vi "In-Context Exit Set Actions-Rev5.vi"(0 "Acquisition Parameters In":T5={"Magnet Angle [deg]"=0.0, "Magnet Angles [deg]"=[], "DeltaVpp [v]"=0.0, "SEM [v]"=0.0, "DeltaVpp Thresh [v]"=0.0, "SEM Thresh [v]"=0.0, "Adaptive Processing"=FALSE, "Acquire Q"=FALSE, "Acquire Photos"=FALSE, "Adaptive Tuning"=FALSE, "Automated Matching"=FALSE, "X-Gradient [G/mm]"=0.0, "Y-Gradient [G/mm]"=0.0, "Z-Gradient [G/mm]"=0.0, "Central Field [G]"=0.0, "Scan Width [G]"=0.0, "Mod. Amp. [G]"=0.0, "Scan Time [s]"=0.0, "Pre-Scan Delay [ms]"=0, "Measurement Timeout [s]"=0.0, "Electromagnet Main Field [G]"=0.0, "Locked Central Field [G]"=0.0, "Scans Excluded"=0, "Scans Completed"=0, "No. Scans/Set"=0, "No. Scans for SNR"=0, "Field Locked Frequency [GHz]"=0.0, "Auto Set-based Field Center"=FALSE, "Prompt for oxy acquisition updates"=FALSE, "Oxy QA Scan?"=FALSE, "Exclude Bad Data"=FALSE, "Optimizing RF Power"=FALSE, "Gradients on/off"=TRUE, "Running Script"=FALSE, "Opto-Coupler Current [A]"=0.0, "Continuous Sweeping"=FALSE, "Sweep Rise Time [sec]"=0, "Reverse Sweep Central Field [G]"=0.0, "Forward Sweep Central Field [G]"=0.0, "Sweep Calibrated"=FALSE, "Modulation Calibrated"=FALSE, "First CheckCal Scan?"=FALSE, "AFC Field Correction"=FALSE, "OxyQAInit Scan Width [G]"=0.0, "OxyQAInit Mod. Amp. [G]"=0.0, "Scans Completed/Session"=0, "Acquire SpO2"=FALSE, "Acquire Temperature"=FALSE, "Over Mod"=FALSE} {"OxyQAInit Mod. Amp. [G]" min=0.0; "OxyQAInit Scan Width [G]" min=0.0; "Mod. Amp. [G]" min=0.0; "Scan Width [G]" min=0.0; "Measurement Timeout [s]" min=0.0; "Scan Time [s]" min=0.0; "Z-Gradient [G/mm]" min=0.0; "Y-Gradient [G/mm]" min=0.0; "X-Gradient [G/mm]" min=0.0; "SEM Thresh [v]" min=0.0; "DeltaVpp Thresh [v]" min=0.0; "SEM [v]" min=0.0}, 5 "Hardware Parameters In":T8={"Scan Calibration [G/V]"=0.0, "Modulation Calibration [G/V]"=0.0, "Modulation Phase [deg]"=0.0, "Modulation Frequency [Hz]"=0.0, "Attenuation [dB]"=0, "Input Channel Count"=0, "Time constant"=7, "Sensitivity"=17, "Frequency Output Voltage [V]"=0.0, "Phase Output Voltage [V]"=0.0, "Lock-in Offset Compensation"=FALSE, "RF [GHz]"=0.0, "Q Start"=0.0, "Q End"=0.0, "Balance"=0.0, "Phase Error"=0.0, "AFC Error"=0.0, "AFC"=FALSE, "Magnet Rotation"=FALSE, "Balance Scaling Factor"=1.0, "Phase Error Scaling Factor"=1.0, "AFC Error Scaling Factor"=1.0, "Frequency Counter ID"="", "Sweep Waveform"=enum."Sawtooth", "Q-Factor Scale"=0.0, " Q-Data Scale"=0.0, " Q-Data Offset"=0.0, "Magnet Rotation Slope"=0.0, "Magnet Rotation Offset"=0.0, "Phase Sweep Resolution"=0.0, "Hardware Version Number"="", "Spectrometer ID Number"=0, "Spectrometer Name"="", "Lock in Saturation"=0.0, "Balance Threshold"=0.0, "Phase Error Threshold"=0.0, "AFC Error Threshold"=0.0, "Linear Actuator Length"=0.0, "Lock-in OK?"=FALSE, "Ignore Lock-in Comm. Failure"=FALSE, "Gradient Addresses"=[], "Gradient Calibrations [G/A*mm]"=[], "Gradient Power Supplies"=[], "Lock-in Address"="", "Magnet Type"=enum."RRI", "Camera Names"=[], "Sweep Limit [Gauss]"=0.0, "Modulation Limit [Gauss]"=0.0, "Balance Threshold Exceeded?"=FALSE, "Phase Threshold Exceeded?"=FALSE, "AFC Threshold Exceeded?"=FALSE, "Consecutive Re-tune attempts"=0, "Reverse Sweep Slope [sec]"=0.0, "Reverse Sweep Offset [G]"=0.0, "AFC Field Correction [V/MHz]"=0.0, "Active Gradients (X Y Z)"=[], "SpO2 Calibration [SpO2/V]"=1.0, "Heart Rate Calibration [BPM/V]"=1.0, "Thermocouple Channel"=""} {"Sensitivity" items=["", "2 nV", "5 nV", "10 nV", "20 nV", "50 nV", "100 nV", "200 nV", "500 nV", "1 uV", "2 uV", "5 uV", "10 uV", "20 uV", "50 uV", "100 uV", "200 uV", "500 uV", "1 mV", "2 mV", "5 mV", "10 mV", "20 mV", "50 mV", "100 mV", "200 mV", "500 mV", "1 V"]; "Time constant" items=["10 us", "20 us", "40 us", "80 us", "160 us", "320 us", "640 us", "5 ms", "10 ms", "20 ms", "50 ms", "100 ms", "200 ms", "500 ms", "1 s", "2 s", "5 s", "10 s", "20 s", "50 s", "100 s", "200 s", "500 s", "1 ks", "2 ks", "5 ks", "10 ks", "20 ks", "50 ks", "100 ks"]}, 9 "Measurement Information In":T1={"Comments"="", "Directory Input"="", "Data file path"=path "C:/Data/EPR Data", "Scripting File"=path "C:/Data/Configuration Script.csv", "Save Data"=FALSE, "Tooth size (d11) [mm]"=0.0, "Tooth size (d12) [mm]"=0.0, "Tooth size (d21) [mm]"=0.0, "Tooth size (d22) [mm]"=0.0, "Dose of Tooth [Gy]"=0.0, "Safe Shutdown?"=FALSE, "Gases Available"=[], "Database Username"="", "Database Password"="", "Database Login URL"="", "Database Upload URL"="", "Database Success URL"="", "Database XML URL"="", "Database Resonator URL"="", "Session Number"=0, "Set #"=0, "Resonator Operator"="", "Session Type"="", "Tooth/Sample ID"="", "Volunteer ID"="", "Computer Operator"="", "Volunteer Type"="", "Site/Tooth Selection (T8,T9)"="", "Resonator"="", "Measurement Site"="", "Non-standard session?"=FALSE, "EPR DAQ Version"="", "Session Path"=path "C:/Data/EPR Data", "Chosen Applied State"="", "Chosen Initial State"="", "Time of Transition"="", "DAQ Mode"=enum."Engineering", "pO2/Scan [mmHg]"=[], "pO2/Set [mmHg]"=[], "Linewidth (HWHM)/Scan [Gauss]"=[], "Linewidth (HWHM)/Set [Gauss]"=[], "pO2 Conversion"="", "Dose Calibration Cluster"={"Dose Response"={"grand_mean"=0.0292016, "slope"=0.0188720543}, "Dose Correction"={"Sex"=1, "a0"=7.719669421, "a1"=-2.746550736, "a2"=-0.186490355, "a3"=0.041922063, "a4"=-0.849147359, "a5"=0.14330063, "a6"=0.019930219, "A_n"=40.0, "H_n"=10.12, "Dose Correction"=FALSE}, "Dose Reporting"={"Reporting is"=TRUE, "sd_threshold [AU]"=0.06, "sd_model [Gy]"=0.66, "dosimetric_threshold [Gy]"=2.0, "Add intrasession errors is"=FALSE, "Prior Radiation?"=FALSE}}, "OxyChip Slope"=0.0, "OxyChip Intercept"=0.0, "QA Mode"=enum."Select QA Mode", "QA Session?"=FALSE, "Sample Type"=enum."Empty Resonator", "Report pO2/Scan"=FALSE, "Skip End Session Save"=FALSE, "Number of sites"=enum."# Probes", "Recipient Name"="", "Sender Name"="", "Recipient Email"="", "Transition State History"=[], "pO2 Report Times"=[], "Temperature [C]"=0.0, "+Error pO2/Scan [mmHg]"=[], "-Error pO2/Scan [mmHg]"=[], "+Error pO2/Set [mmHg]"=[], "-Error pO2/Set [mmHg]"=[], "Oxy Phase Exclusion Tolerance [rad]"=0.0, "Oxy Center Exclusion Tolerance [%]"=0.0, "Oxy Exclude Unacceptable"=FALSE, "Oxy Unacceptable Estimate Flags"=[], "Save Session PPT"=FALSE, "Flagged Bad Sets"=[]} {"Oxy Center Exclusion Tolerance [%]" format="%#_9g"; "Oxy Phase Exclusion Tolerance [rad]" format="%#_9g"; "Temperature [C]" format="%#_9g"; "OxyChip Intercept" format="%#_9g"; "OxyChip Slope" format="%#_9g"; "Dose Calibration Cluster"."Dose Reporting"."dosimetric_threshold [Gy]" format="%#_9g"; "Dose Calibration Cluster"."Dose Reporting"."sd_model [Gy]" format="%#_9g"; "Dose Calibration Cluster"."Dose Reporting"."sd_threshold [AU]" format="%#_9g"; "Dose Calibration Cluster"."Dose Correction"."H_n" format="%#_9g"; "Dose Calibration Cluster"."Dose Correction"."A_n" format="%#_9g"; "Dose Calibration Cluster"."Dose Correction"."a6" format="%#.9g"; "Dose Calibration Cluster"."Dose Correction"."a5" format="%#.9g"; "Dose Calibration Cluster"."Dose Correction"."a4" format="%#.9g"; "Dose Calibration Cluster"."Dose Correction"."a3" format="%#.9g"; "Dose Calibration Cluster"."Dose Correction"."a2" format="%#.9g"; "Dose Calibration Cluster"."Dose Correction"."a1" format="%#.9g"; "Dose Calibration Cluster"."Dose Correction"."a0" format="%#.9g"; "Dose Calibration Cluster"."Dose Correction"."Sex" items=["Male"=1, "Female"=0]; "Dose Calibration Cluster"."Dose Response"."slope" format="%#_9g"; "Dose Calibration Cluster"."Dose Response"."grand_mean" format="%#_9g"}, 11 "Spectral Data In":T6={"PDT Amp [v]"=0.0, "RIS Amp [v]"=0.0, "B-Field"=[], "All In-Phase Scan Spectra"=[], "Model Select"=enum."OneCompRISTwoPDT", "Fit Each Scan"=FALSE, "PDT Center [g]"=0.0, "In-Phase Average Spectra"=[], "In-Phase Median Spectra"=[], "Out-Phase Median Spectra"=[], "Out-Phase Average Spectra"=[], "Fit Spectra"=[], "Fit No-Baseline Spectra"=[], "All Out-Phase Scan Spectra"=[], "Baseline Offset Correction"=FALSE, "In-Phase Offset [v]"=0.0, "Out-Phase Offset [v]"=0.0, "Ch2 Input\n(Balance)"=[], "Ch3 Input\n(Phase)"=[], "Ch4 Input\n(AFC)"=[], "Fit Pars"=[], "Fit Pars Errors"=[], "Fit Pars Labels"=[], "Raw Scan DAQ Data"=[], "Bad Scans Indicies"=[], "Good In-Phase Scan Spectra"=[], "Good Out-Phase Scan Spectra"=[], "Bad In-Phase Scan Spectra"=[], "Bad Out-Phase Scan Spectra"=[], "Number of bad scans"=0, "Fit History"=[], "PDT Amp. History/Set [v]"=[], "RIS Amp. History/Set [v]"=[], "RIS Amp. History/Scan [v]"=[], "All Shifted B-Fields"=[], "Good Shifted B-Fields"=[], "Ch5 Input\n(SpO2)"=[], "Ch6 Input\n(BPM)"=[], "Global SNR"=0.0, "Fit Error History"=[], "SNR History"=[]} {"Global SNR" min=0.0; "PDT Center [g]" min=0.0; "RIS Amp [v]" min=0.0; "PDT Amp [v]" min=0.0}) -> (1 "Exclude pO2 Estimate":bool, 2 "Scan Width [G]":dbl, 3 "Mod. Amp. [G]":dbl, 4 "Acquisition Parameters Out":T5={"Magnet Angle [deg]"=0.0, "Magnet Angles [deg]"=[], "DeltaVpp [v]"=0.0, "SEM [v]"=0.0, "DeltaVpp Thresh [v]"=0.0, "SEM Thresh [v]"=0.0, "Adaptive Processing"=FALSE, "Acquire Q"=FALSE, "Acquire Photos"=FALSE, "Adaptive Tuning"=FALSE, "Automated Matching"=FALSE, "X-Gradient [G/mm]"=0.0, "Y-Gradient [G/mm]"=0.0, "Z-Gradient [G/mm]"=0.0, "Central Field [G]"=0.0, "Scan Width [G]"=0.0, "Mod. Amp. [G]"=0.0, "Scan Time [s]"=0.0, "Pre-Scan Delay [ms]"=0, "Measurement Timeout [s]"=0.0, "Electromagnet Main Field [G]"=0.0, "Locked Central Field [G]"=0.0, "Scans Excluded"=0, "Scans Completed"=0, "No. Scans/Set"=0, "No. Scans for SNR"=0, "Field Locked Frequency [GHz]"=0.0, "Auto Set-based Field Center"=FALSE, "Prompt for oxy acquisition updates"=FALSE, "Oxy QA Scan?"=FALSE, "Exclude Bad Data"=FALSE, "Optimizing RF Power"=FALSE, "Gradients on/off"=TRUE, "Running Script"=FALSE, "Opto-Coupler Current [A]"=0.0, "Continuous Sweeping"=FALSE, "Sweep Rise Time [sec]"=0, "Reverse Sweep Central Field [G]"=0.0, "Forward Sweep Central Field [G]"=0.0, "Sweep Calibrated"=FALSE, "Modulation Calibrated"=FALSE, "First CheckCal Scan?"=FALSE, "AFC Field Correction"=FALSE, "OxyQAInit Scan Width [G]"=0.0, "OxyQAInit Mod. Amp. [G]"=0.0, "Scans Completed/Session"=0, "Acquire SpO2"=FALSE, "Acquire Temperature"=FALSE, "Over Mod"=FALSE} {"OxyQAInit Mod. Amp. [G]" min=0.0; "OxyQAInit Scan Width [G]" min=0.0; "Mod. Amp. [G]" min=0.0; "Scan Width [G]" min=0.0; "Measurement Timeout [s]" min=0.0; "Scan Time [s]" min=0.0; "Z-Gradient [G/mm]" min=0.0; "Y-Gradient [G/mm]" min=0.0; "X-Gradient [G/mm]" min=0.0; "SEM Thresh [v]" min=0.0; "DeltaVpp Thresh [v]" min=0.0; "SEM [v]" min=0.0}, 6 "Measurement Information Out":T1={"Comments"="", "Directory Input"="", "Data file path"=path "C:/Data/EPR Data", "Scripting File"=path "C:/Data/Configuration Script.csv", "Save Data"=FALSE, "Tooth size (d11) [mm]"=0.0, "Tooth size (d12) [mm]"=0.0, "Tooth size (d21) [mm]"=0.0, "Tooth size (d22) [mm]"=0.0, "Dose of Tooth [Gy]"=0.0, "Safe Shutdown?"=FALSE, "Gases Available"=[], "Database Username"="", "Database Password"="", "Database Login URL"="", "Database Upload URL"="", "Database Success URL"="", "Database XML URL"="", "Database Resonator URL"="", "Session Number"=0, "Set #"=0, "Resonator Operator"="", "Session Type"="", "Tooth/Sample ID"="", "Volunteer ID"="", "Computer Operator"="", "Volunteer Type"="", "Site/Tooth Selection (T8,T9)"="", "Resonator"="", "Measurement Site"="", "Non-standard session?"=FALSE, "EPR DAQ Version"="", "Session Path"=path "C:/Data/EPR Data", "Chosen Applied State"="", "Chosen Initial State"="", "Time of Transition"="", "DAQ Mode"=enum."Engineering", "pO2/Scan [mmHg]"=[], "pO2/Set [mmHg]"=[], "Linewidth (HWHM)/Scan [Gauss]"=[], "Linewidth (HWHM)/Set [Gauss]"=[], "pO2 Conversion"="", "Dose Calibration Cluster"={"Dose Response"={"grand_mean"=0.0292016, "slope"=0.0188720543}, "Dose Correction"={"Sex"=1, "a0"=7.719669421, "a1"=-2.746550736, "a2"=-0.186490355, "a3"=0.041922063, "a4"=-0.849147359, "a5"=0.14330063, "a6"=0.019930219, "A_n"=40.0, "H_n"=10.12, "Dose Correction"=FALSE}, "Dose Reporting"={"Reporting is"=TRUE, "sd_threshold [AU]"=0.06, "sd_model [Gy]"=0.66, "dosimetric_threshold [Gy]"=2.0, "Add intrasession errors is"=FALSE, "Prior Radiation?"=FALSE}}, "OxyChip Slope"=0.0, "OxyChip Intercept"=0.0, "QA Mode"=enum."Select QA Mode", "QA Session?"=FALSE, "Sample Type"=enum."Empty Resonator", "Report pO2/Scan"=FALSE, "Skip End Session Save"=FALSE, "Number of sites"=enum."# Probes", "Recipient Name"="", "Sender Name"="", "Recipient Email"="", "Transition State History"=[], "pO2 Report Times"=[], "Temperature [C]"=0.0, "+Error pO2/Scan [mmHg]"=[], "-Error pO2/Scan [mmHg]"=[], "+Error pO2/Set [mmHg]"=[], "-Error pO2/Set [mmHg]"=[], "Oxy Phase Exclusion Tolerance [rad]"=0.0, "Oxy Center Exclusion Tolerance [%]"=0.0, "Oxy Exclude Unacceptable"=FALSE, "Oxy Unacceptable Estimate Flags"=[], "Save Session PPT"=FALSE, "Flagged Bad Sets"=[]} {"Oxy Center Exclusion Tolerance [%]" format="%#_9g"; "Oxy Phase Exclusion Tolerance [rad]" format="%#_9g"; "Temperature [C]" format="%#_9g"; "OxyChip Intercept" format="%#_9g"; "OxyChip Slope" format="%#_9g"; "Dose Calibration Cluster"."Dose Reporting"."dosimetric_threshold [Gy]" format="%#_9g"; "Dose Calibration Cluster"."Dose Reporting"."sd_model [Gy]" format="%#_9g"; "Dose Calibration Cluster"."Dose Reporting"."sd_threshold [AU]" format="%#_9g"; "Dose Calibration Cluster"."Dose Correction"."H_n" format="%#_9g"; "Dose Calibration Cluster"."Dose Correction"."A_n" format="%#_9g"; "Dose Calibration Cluster"."Dose Correction"."a6" format="%#.9g"; "Dose Calibration Cluster"."Dose Correction"."a5" format="%#.9g"; "Dose Calibration Cluster"."Dose Correction"."a4" format="%#.9g"; "Dose Calibration Cluster"."Dose Correction"."a3" format="%#.9g"; "Dose Calibration Cluster"."Dose Correction"."a2" format="%#.9g"; "Dose Calibration Cluster"."Dose Correction"."a1" format="%#.9g"; "Dose Calibration Cluster"."Dose Correction"."a0" format="%#.9g"; "Dose Calibration Cluster"."Dose Correction"."Sex" items=["Male"=1, "Female"=0]; "Dose Calibration Cluster"."Dose Response"."slope" format="%#_9g"; "Dose Calibration Cluster"."Dose Response"."grand_mean" format="%#_9g"}, 8 "Spectral Data Out":T6={"PDT Amp [v]"=0.0, "RIS Amp [v]"=0.0, "B-Field"=[], "All In-Phase Scan Spectra"=[], "Model Select"=enum."OneCompRISTwoPDT", "Fit Each Scan"=FALSE, "PDT Center [g]"=0.0, "In-Phase Average Spectra"=[], "In-Phase Median Spectra"=[], "Out-Phase Median Spectra"=[], "Out-Phase Average Spectra"=[], "Fit Spectra"=[], "Fit No-Baseline Spectra"=[], "All Out-Phase Scan Spectra"=[], "Baseline Offset Correction"=FALSE, "In-Phase Offset [v]"=0.0, "Out-Phase Offset [v]"=0.0, "Ch2 Input\n(Balance)"=[], "Ch3 Input\n(Phase)"=[], "Ch4 Input\n(AFC)"=[], "Fit Pars"=[], "Fit Pars Errors"=[], "Fit Pars Labels"=[], "Raw Scan DAQ Data"=[], "Bad Scans Indicies"=[], "Good In-Phase Scan Spectra"=[], "Good Out-Phase Scan Spectra"=[], "Bad In-Phase Scan Spectra"=[], "Bad Out-Phase Scan Spectra"=[], "Number of bad scans"=0, "Fit History"=[], "PDT Amp. History/Set [v]"=[], "RIS Amp. History/Set [v]"=[], "RIS Amp. History/Scan [v]"=[], "All Shifted B-Fields"=[], "Good Shifted B-Fields"=[], "Ch5 Input\n(SpO2)"=[], "Ch6 Input\n(BPM)"=[], "Global SNR"=0.0, "Fit Error History"=[], "SNR History"=[]} {"Global SNR" min=0.0; "PDT Center [g]" min=0.0; "RIS Amp [v]" min=0.0; "PDT Amp [v]" min=0.0}, 10 "QSM Response":cluster{"Enum":T4, "Data":variant}[](array[cluster]), 12 "Magnet Angle [deg]":dbl, 13 "Calibration dBpp/Set [Gauss]":dbl[][](array[numeric]), 14 "pO2/Set [mmHg]":dbl[][](array[numeric]), 15 "error out":errorcluster)   [LabVIEW 2016]
uses:
  Types/Acquisition Parameters.ctl
  Types/Hardware Parameters.ctl
  Types/Measurement Information.ctl
  Analysis/Dose Calculation and Reporting/Dose Calculation Control.ctl
  Types/Sample Type.ctl
  Types/Spectral Data.ctl
  Types/Fitting Model Selection.ctl
  Types/State Control.ctl
  Types/Global Variables.vi
panel:
  # "Session Information"
  # "Oximetric Data and Information"
  # "Email"
  # "Tooth Information"
  # "Database"
  # "Gradients"
  # "Field"
  # "Scans and Sets"
  # "Timing"
  # "Adaptive Dosimetric \nData Processing"
  # "Session Information"
  # "Oximetric Data and Information"
  # "Email"
  # "Tooth Information"
  # "Database"
  # "Bridge I/O"
  # "Magnet Rotation"
  # "Field Calibration"
  # "Lock In Amplifier"
  # "Spectrometer Information"
  # "DAQ Settings"
  # "Gradient Coils and Field"
  # "X"
  # "Y"
  # "Z"
  # "Q-Measurements"
  # "Gradients"
  # "Field"
  # "Scans and Sets"
  # "Timing"
  # "Adaptive Dosimetric \nData Processing"
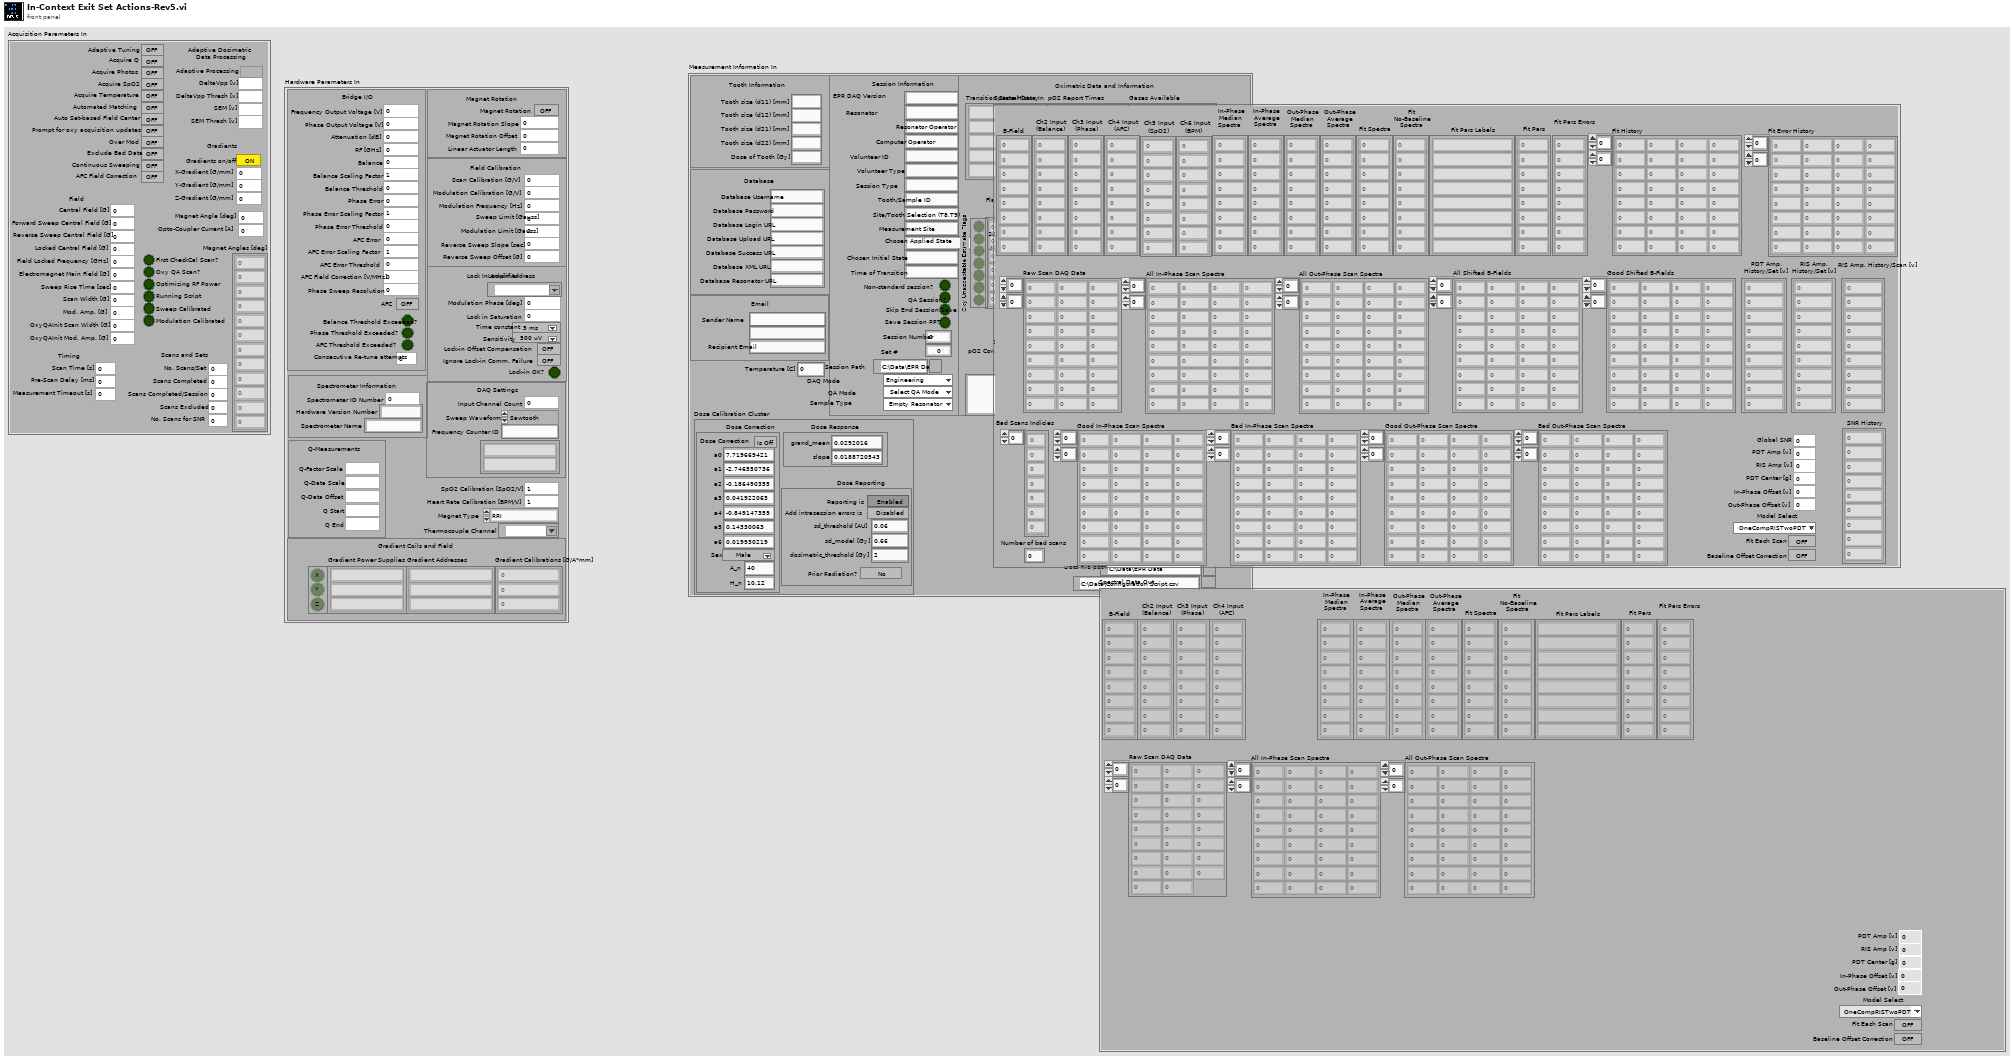
[diagram p1: front panel]
types:
  T1 = typedef "Measurement Information.ctl" = cluster{"Comments":string, "Directory Input":string, "Data file path":path, "Scripting File":path, "Save Data":bool, "Tooth size (d11) [mm]":dbl, "Tooth size (d12) [mm]":dbl, "Tooth size (d21) [mm]":dbl, "Tooth size (d22) [mm]":dbl, "Dose of Tooth [Gy]":dbl, "Safe Shutdown?":bool, "Gases Available":string[], "Database Username":string, "Database Password":string, "Database Login URL":string, "Database Upload URL":string, "Database Success URL":string, "Database XML URL":string, "Database Resonator URL":string, "Session Number":i32, "Set #":u32, "Resonator Operator":string, "Session Type":string, "Tooth/Sample ID":string, "Volunteer ID":string, "Computer Operator":string, "Volunteer Type":string, "Site/Tooth Selection (T8,T9)":string, "Resonator":string, "Measurement Site":string, "Non-standard session?":bool, "EPR DAQ Version":string, "Session Path":path, "Chosen Applied State":string, "Chosen Initial State":string, "Time of Transition":string, "DAQ Mode":enum16{"Engineering", "Dosimetry", "Oximetry"}, "pO2/Scan [mmHg]":dbl[][], "pO2/Set [mmHg]":dbl[][], "Linewidth (HWHM)/Scan [Gauss]":dbl[][], "Linewidth (HWHM)/Set [Gauss]":dbl[][], "pO2 Conversion":string, "Dose Calibration Cluster":T2, "OxyChip Slope":dbl, "OxyChip Intercept":dbl, "QA Mode":enum16{"Select QA Mode", "QA-Start/End", "QA-Mid", "QA-Weekly", "QA-Eng", "Check Calibration"}, "QA Session?":bool, "Sample Type":T3, "Report pO2/Scan":bool, "Skip End Session Save":bool, "Number of sites":enum16{"# Probes", "1", "2", "3", "4"}, "Recipient Name":string, "Sender Name":string, "Recipient Email":string, "Transition State History":string[], "pO2 Report Times":string[], "Temperature [C]":dbl, "+Error pO2/Scan [mmHg]":dbl[][], "-Error pO2/Scan [mmHg]":dbl[][], "+Error pO2/Set [mmHg]":dbl[][], "-Error pO2/Set [mmHg]":dbl[][], "Oxy Phase Exclusion Tolerance [rad]":dbl, "Oxy Center Exclusion Tolerance [%]":dbl, "Oxy Exclude Unacceptable":bool, "Oxy Unacceptable Estimate Flags":bool[], "Save Session PPT":bool, "Flagged Bad Sets":u32[]}
  T2 = typedef "Dose Calculation Control.ctl" = cluster{"Dose Response":cluster{"grand_mean":dbl, "slope":dbl}, "Dose Correction":cluster{"Sex":u16, "a0":dbl, "a1":dbl, "a2":dbl, "a3":dbl, "a4":dbl, "a5":dbl, "a6":dbl, "A_n":dbl, "H_n":dbl, "Dose Correction":bool}, "Dose Reporting":cluster{"Reporting is":bool, "sd_threshold [AU]":dbl, "sd_model [Gy]":dbl, "dosimetric_threshold [Gy]":dbl, "Add intrasession errors is":bool, "Prior Radiation?":bool}}
  T3 = typedef "Sample Type.ctl" = enum16{"Empty Resonator", "IRS", "BallZero", "Irradiated Tooth", "Non-irradiated Tooth", "OxyChip", "LiPc", "PDT", "India Ink"}
  T4 = typedef "State Control.ctl" = enum16{"Startup", "Read Config File", "Initilize Optional Hardware", "Idle", "New Session", "Read GUI Pars", "Configure Hardware", "Initialize Set", "Pre-Scan", "Scan", "Post-Scan", "Exit Set", "Automated Tuning", "Manual Tuning", "Check Calibration", "Optimize RF Power", "Test Scan", "Set Oxy QA-Scan Pars", "Find Peaks", "Update from Cursors", "Flag Bad Set", "Mark transition time", "Measure Q", "Measure Noise", "Rotate Magnet", "Lock Field", "Engineering Tuning", "Zero Voltages", "Update Center Field", "Refit Data", "Open Session Data Folder", "AfterSave", "Undo Auto Update Pars", "Read from Script", "End Session", "Quit Software", "Error"}
  T5 = typedef "Acquisition Parameters.ctl" = cluster{"Magnet Angle [deg]":dbl, "Magnet Angles [deg]":dbl[], "DeltaVpp [v]":dbl, "SEM [v]":dbl, "DeltaVpp Thresh [v]":dbl, "SEM Thresh [v]":dbl, "Adaptive Processing":bool, "Acquire Q":bool, "Acquire Photos":bool, "Adaptive Tuning":bool, "Automated Matching":bool, "X-Gradient [G/mm]":dbl, "Y-Gradient [G/mm]":dbl, "Z-Gradient [G/mm]":dbl, "Central Field [G]":dbl, "Scan Width [G]":dbl, "Mod. Amp. [G]":dbl, "Scan Time [s]":dbl, "Pre-Scan Delay [ms]":u32, "Measurement Timeout [s]":dbl, "Electromagnet Main Field [G]":dbl, "Locked Central Field [G]":dbl, "Scans Excluded":u32, "Scans Completed":u32, "No. Scans/Set":u32, "No. Scans for SNR":u32, "Field Locked Frequency [GHz]":dbl, "Auto Set-based Field Center":bool, "Prompt for oxy acquisition updates":bool, "Oxy QA Scan?":bool, "Exclude Bad Data":bool, "Optimizing RF Power":bool, "Gradients on/off":bool, "Running Script":bool, "Opto-Coupler Current [A]":dbl, "Continuous Sweeping":bool, "Sweep Rise Time [sec]":u32, "Reverse Sweep Central Field [G]":dbl, "Forward Sweep Central Field [G]":dbl, "Sweep Calibrated":bool, "Modulation Calibrated":bool, "First CheckCal Scan?":bool, "AFC Field Correction":bool, "OxyQAInit Scan Width [G]":dbl, "OxyQAInit Mod. Amp. [G]":dbl, "Scans Completed/Session":u32, "Acquire SpO2":bool, "Acquire Temperature":bool, "Over Mod":bool}
  T6 = typedef "Spectral Data.ctl" = cluster{"PDT Amp [v]":dbl, "RIS Amp [v]":dbl, "B-Field":dbl[], "All In-Phase Scan Spectra":dbl[][], "Model Select":T7, "Fit Each Scan":bool, "PDT Center [g]":dbl, "In-Phase Average Spectra":dbl[], "In-Phase Median Spectra":dbl[], "Out-Phase Median Spectra":dbl[], "Out-Phase Average Spectra":dbl[], "Fit Spectra":dbl[], "Fit No-Baseline Spectra":dbl[], "All Out-Phase Scan Spectra":dbl[][], "Baseline Offset Correction":bool, "In-Phase Offset [v]":dbl, "Out-Phase Offset [v]":dbl, "Ch2 Input\n(Balance)":dbl[], "Ch3 Input\n(Phase)":dbl[], "Ch4 Input\n(AFC)":dbl[], "Fit Pars":dbl[], "Fit Pars Errors":dbl[], "Fit Pars Labels":string[], "Raw Scan DAQ Data":dbl[][], "Bad Scans Indicies":i32[], "Good In-Phase Scan Spectra":dbl[][], "Good Out-Phase Scan Spectra":dbl[][], "Bad In-Phase Scan Spectra":dbl[][], "Bad Out-Phase Scan Spectra":dbl[][], "Number of bad scans":i32, "Fit History":dbl[][], "PDT Amp. History/Set [v]":dbl[], "RIS Amp. History/Set [v]":dbl[], "RIS Amp. History/Scan [v]":dbl[], "All Shifted B-Fields":dbl[][], "Good Shifted B-Fields":dbl[][], "Ch5 Input\n(SpO2)":dbl[], "Ch6 Input\n(BPM)":dbl[], "Global SNR":dbl, "Fit Error History":dbl[][], "SNR History":dbl[]}
  T7 = typedef "Fitting Model Selection.ctl" = enum16{"OneCompRIS", "OneCompRISTwoPDT", "OneCompRISRev", "OneCompRISTwoPDTRev", "LiPc", "TwoLiPc", "ThreeLiPc", "FourLiPc", "PDTCalibration", "CE_Ink", "Printex", "MelaninTwoPDT"}
  T8 = typedef "Hardware Parameters.ctl" = cluster{"Scan Calibration [G/V]":dbl, "Modulation Calibration [G/V]":dbl, "Modulation Phase [deg]":dbl, "Modulation Frequency [Hz]":dbl, "Attenuation [dB]":u16, "Input Channel Count":i32, "Time constant":u16, "Sensitivity":u16, "Frequency Output Voltage [V]":dbl, "Phase Output Voltage [V]":dbl, "Lock-in Offset Compensation":bool, "RF [GHz]":dbl, "Q Start":dbl, "Q End":dbl, "Balance":dbl, "Phase Error":dbl, "AFC Error":dbl, "AFC":bool, "Magnet Rotation":bool, "Balance Scaling Factor":dbl, "Phase Error Scaling Factor":dbl, "AFC Error Scaling Factor":dbl, "Frequency Counter ID":string, "Sweep Waveform":enum16{"Sine Wave", "Square Wave", "Sawtooth", "Triangle Wave"}, "Q-Factor Scale":dbl, " Q-Data Scale":dbl, " Q-Data Offset":dbl, "Magnet Rotation Slope":dbl, "Magnet Rotation Offset":dbl, "Phase Sweep Resolution":dbl, "Hardware Version Number":string, "Spectrometer ID Number":i32, "Spectrometer Name":string, "Lock in Saturation":dbl, "Balance Threshold":dbl, "Phase Error Threshold":dbl, "AFC Error Threshold":dbl, "Linear Actuator Length":dbl, "Lock-in OK?":bool, "Ignore Lock-in Comm. Failure":bool, "Gradient Addresses":string[], "Gradient Calibrations [G/A*mm]":dbl[], "Gradient Power Supplies":string[], "Lock-in Address":refnum<visa-resource-name>, "Magnet Type":enum16{"RRI", "BARDA", "Whole Body Permanent", "RRI Electromagnet"}, "Camera Names":string[], "Sweep Limit [Gauss]":dbl, "Modulation Limit [Gauss]":dbl, "Balance Threshold Exceeded?":bool, "Phase Threshold Exceeded?":bool, "AFC Threshold Exceeded?":bool, "Consecutive Re-tune attempts":i32, "Reverse Sweep Slope [sec]":dbl, "Reverse Sweep Offset [G]":dbl, "AFC Field Correction [V/MHz]":dbl, "Active Gradients (X Y Z)":bool[], "SpO2 Calibration [SpO2/V]":dbl, "Heart Rate Calibration [BPM/V]":dbl, "Thermocouple Channel":tag}
  T9 = enum16{"Select QA Mode", "QA-Start/End", "QA-Mid", "QA-Weekly", "QA-Eng", "Check Calibration"}
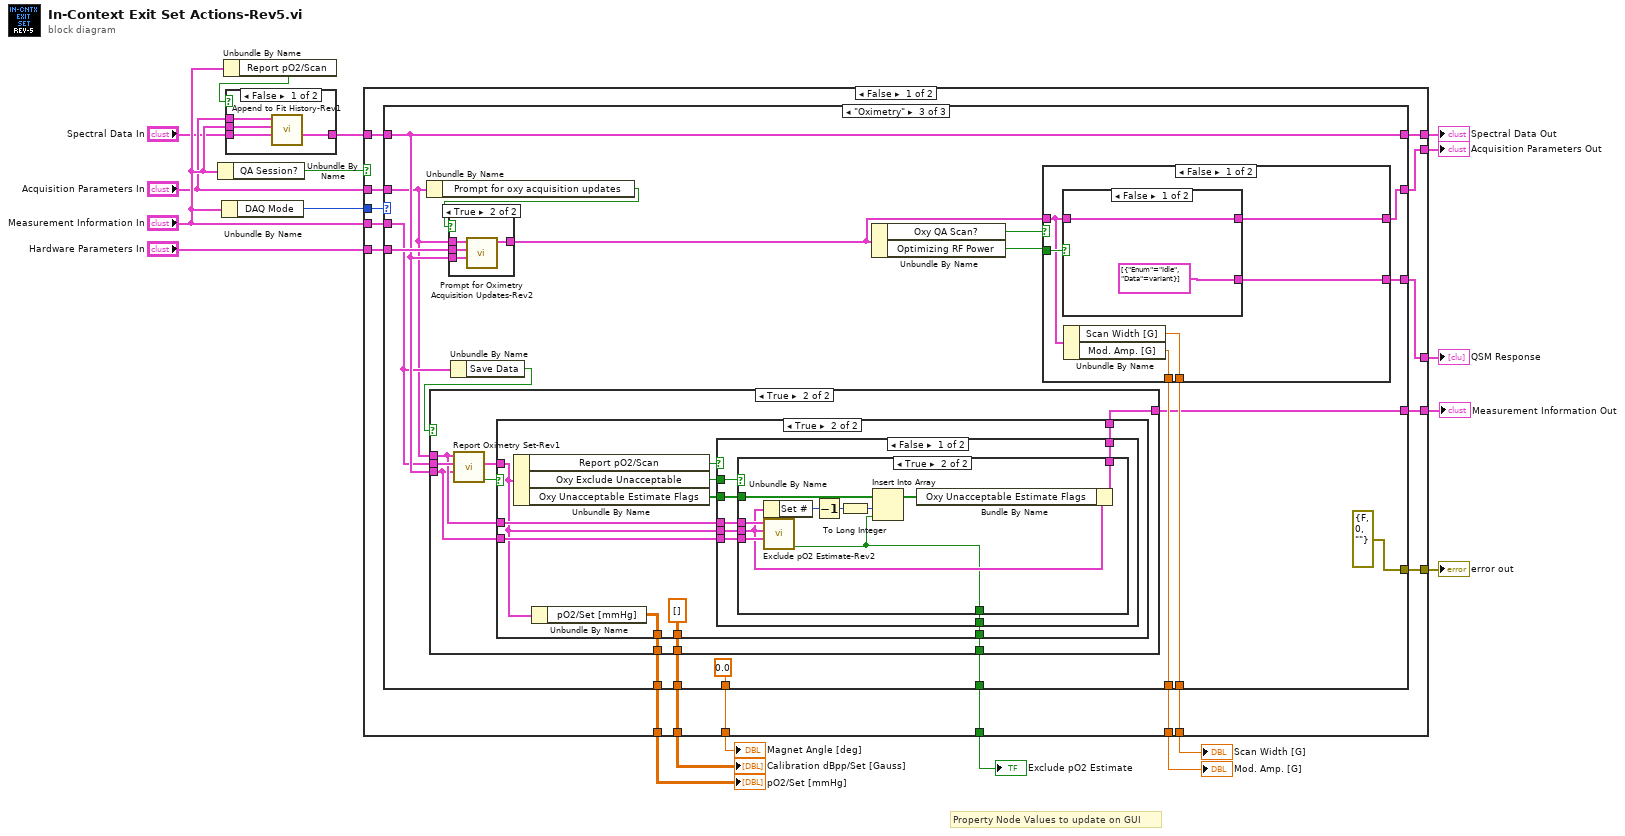
[diagram p0: block diagram]
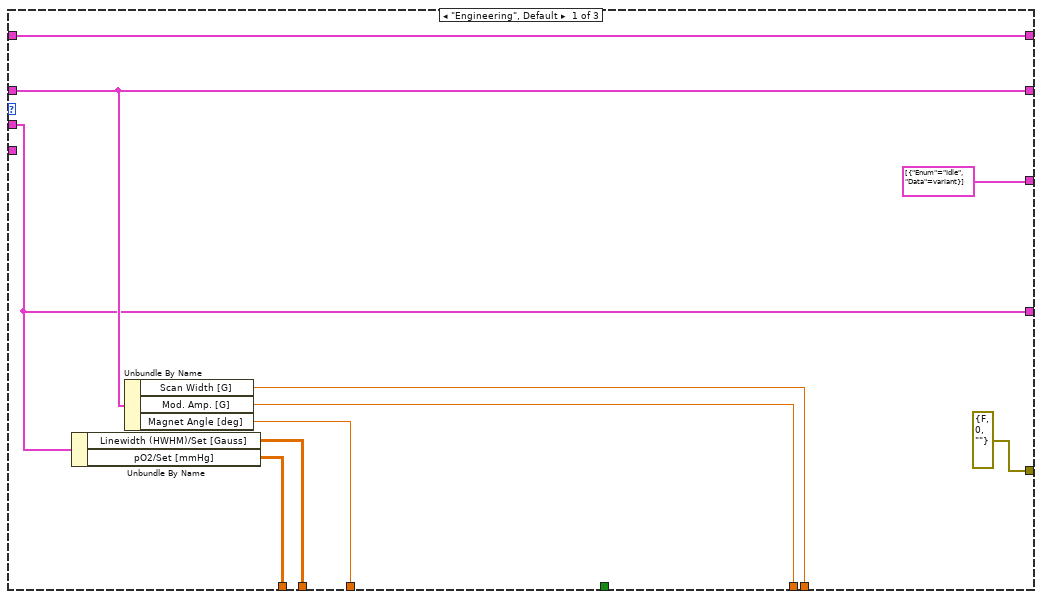
[diagram p3: hidden frame]
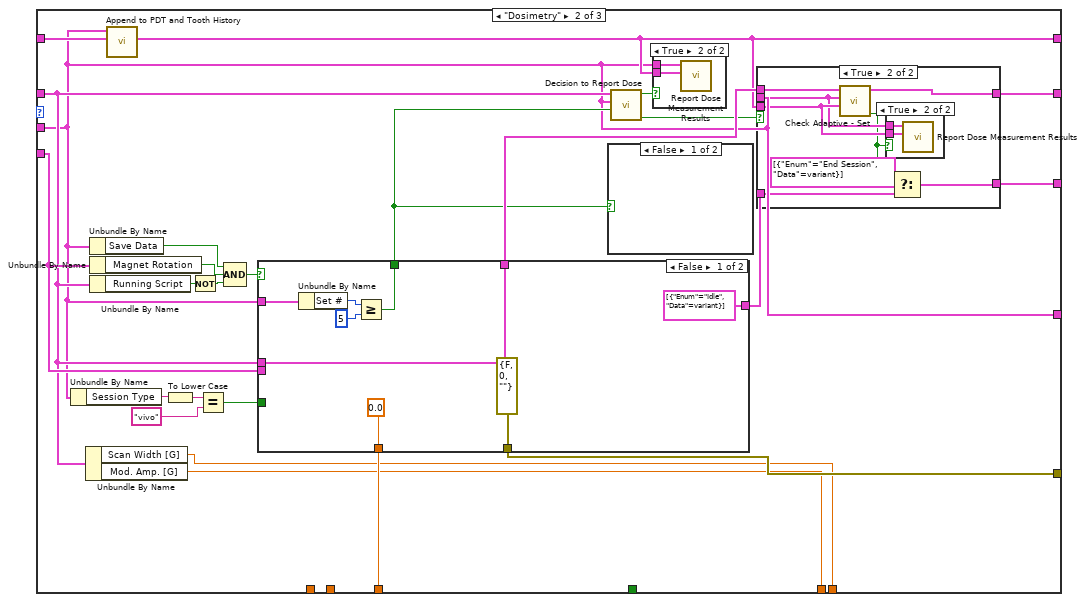
[diagram p4: hidden frame]
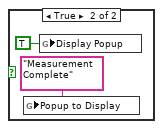
[diagram p5: hidden frame]
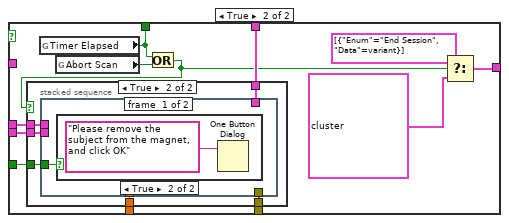
[diagram p9: hidden frame]
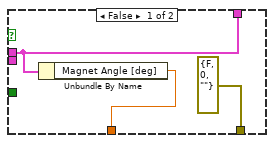
[diagram p10: hidden frame]
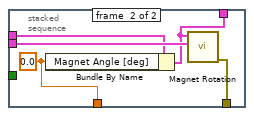
[diagram p12: hidden frame]
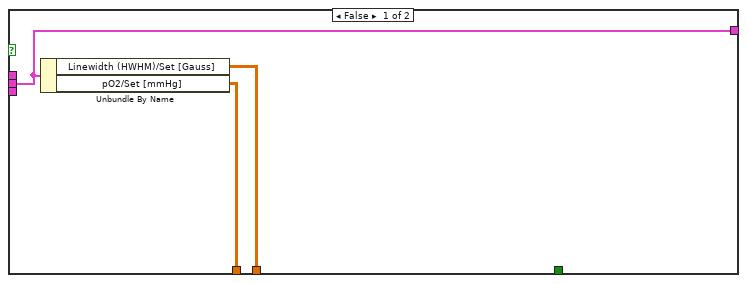
[diagram p13: hidden frame]
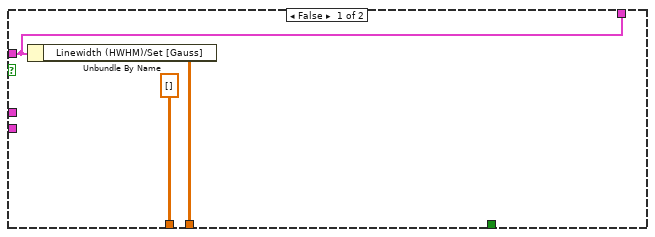
[diagram p14: hidden frame]
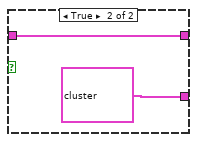
[diagram p17: hidden frame]
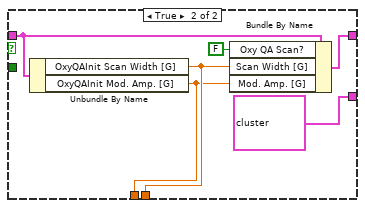
[diagram p18: hidden frame]
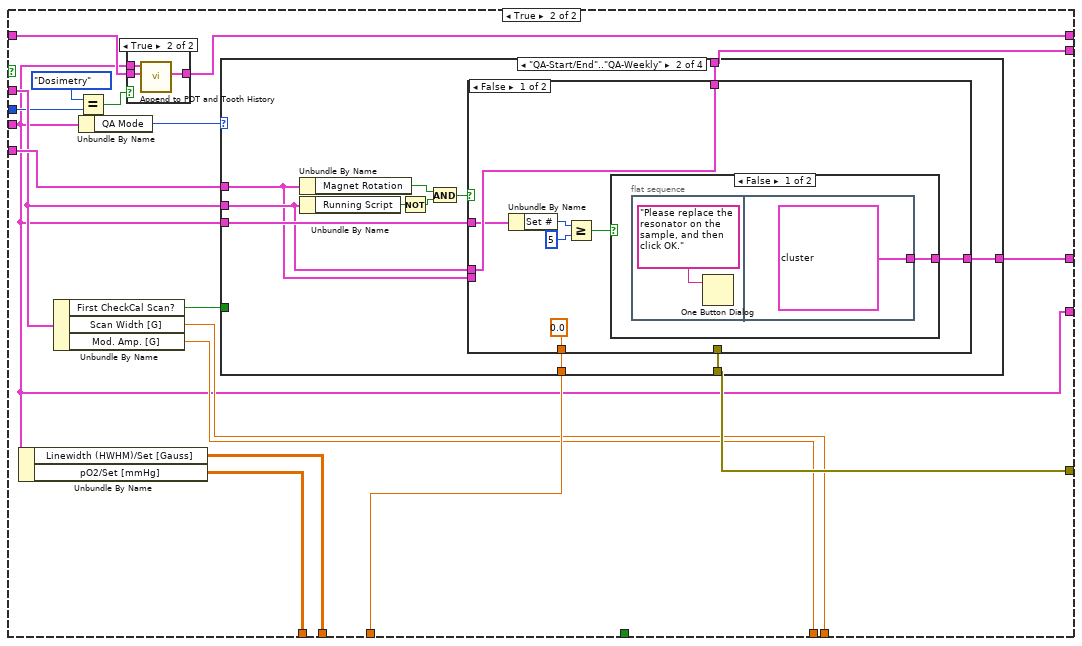
[diagram p20: hidden frame]
diagram:
  # "Property Node Values to update on GUI"
  n1 = Unbundle By Name("Measurement Information In") -> ("QA Session?"=w10:bool)
  n2 = Unbundle By Name("Measurement Information In") -> ("DAQ Mode"=w19:enum16{"Engineering", "Dosimetry", "Oximetry"})
  n3 = Unbundle By Name("Measurement Information In") -> ("Report pO2/Scan"=w6:bool)
  n4 = case shown="False" w6 {
    tunnel: "Measurement Information In" -> [w23 _]
    tunnel: "Spectral Data In" -> [w22 w24]
    tunnel: "Acquisition Parameters In" -> [w21 _]
    tunnel: [w20 w24] -> w2
    frame False {
      n5 = call "Append to Fit History-Rev1.vi"("Spectral Data In"=w22, "Measurement Information In"=w23, "Acquisition Parameters"=w21) -> ("Spectral Data Out"=w20:T6)  [unwired: 6 in]
    }
    frame True {
    }
  }
  n6 = case shown="False" w10 {
    tunnel: w19 -> [w40 w219]
    tunnel: "Acquisition Parameters In" -> [w39 w223]
    tunnel: "Hardware Parameters In" -> [w38 w224]
    tunnel: w2 -> [w37 w216]
    tunnel: [w36 w222] -> w17
    tunnel: [w35 w215] -> w16
    tunnel: [w34 w226] -> w15
    tunnel: [w33 w229] -> w14
    tunnel: [w32 w228] -> w13
    tunnel: [w31 w220] -> w12
    tunnel: [w30 w221] -> w11
    tunnel: "Measurement Information In" -> [w29 w212]
    tunnel: [w28 w214] -> w9
    tunnel: [w27 w213] -> w8
    tunnel: [w26 w212] -> w7
    tunnel: [w25 _] -> w1
    frame False {
      n7 = case shown="\"Oximetry\"" w40 {
        tunnel: w39 -> [w47 w54 w130]
        tunnel: w38 -> [_ w74 w146]
        tunnel: w37 -> [w49 w75 w141]
        tunnel: w29 -> [w41 w51 w135]
        tunnel: [cluster{"Enum":T4, "Data":variant}[] [{"Enum"=enum."Idle", "Data"=variant}] w71 w142] -> w34
        tunnel: [w49 w69 w141] -> w35
        tunnel: [errorcluster {"status"=FALSE, "code"=0, "source"=""} ("error out") w73 errorcluster {"status"=FALSE, "code"=0, "source"=""} ("error out")] -> w30
        tunnel: [w47 w68 w139] -> w36
        tunnel: [w44 _ w138] -> w33
        tunnel: [w45 _ w137] -> w32
        tunnel: [w46 w61 0.0 ("Magnet Angle [deg]")] -> w31
        tunnel: [w43 w53 w132] -> w28
        tunnel: [w42 w52 w131] -> w27
        tunnel: [w41 w51 w129] -> w26
        tunnel: [_ _ w128] -> w25
        frame "Engineering", Default {
          n8 = Unbundle By Name(w41) -> ("Linewidth (HWHM)/Set [Gauss]"=w45:dbl[][], "pO2/Set [mmHg]"=w44:dbl[][])
          n9 = Unbundle By Name(w47) -> ("Scan Width [G]"=w43:dbl, "Mod. Amp. [G]"=w42:dbl, "Magnet Angle [deg]"=w46:dbl)
        }
        frame "Dosimetry" {
          n10 = Unbundle By Name(w51) -> ("Session Type"=w57:string)
          n11 = Unbundle By Name(w54) -> ("Scan Width [G]"=w53:dbl, "Mod. Amp. [G]"=w52:dbl)
          n12 = Unbundle By Name(w51) -> ("Save Data"=w55:bool)
          n13 = Unbundle By Name(w74) -> ("Magnet Rotation"=w65:bool)
          n14 = Unbundle By Name(w54) -> ("Running Script"=w67:bool)
          n15 = call "Append to PDT and Tooth History.vi"("Spectral Data In"=w75, "Measurement Information In"=w51) -> ("Spectral Data Out"=w69:T6)  [unwired: 9 in]
          n16 = To Lower Case(string=w57) -> (all lower case string=w58:string)
          n17 = Not(x=w67) -> (.not. x?=w66:bool)
          n18 = Equal?(x=w58, y="vivo" ("Session Type")) -> (x = y?=w56:bool)
          n19 = Compound Arithmetic op=AND(w55, w65, w66) -> (w64:bool)
          n20 = case shown="False" w64 {
            tunnel: [cluster{"Enum":T4, "Data":variant}[] [{"Enum"=enum."Idle", "Data"=variant}] w109] -> w72
            tunnel: w54 -> [w98 w108]
            tunnel: w74 -> [_ w107]
            tunnel: [w98 w106] -> w70
            tunnel: [errorcluster {"status"=FALSE, "code"=0, "source"=""} ("error out") w105] -> w73
            tunnel: [w96 w102] -> w60
            tunnel: w51 -> [w93 _]
            tunnel: [0.0 ("Magnet Angle [deg]") w101] -> w61
            tunnel: w56 -> [_ w100]
            frame False {
              n21 = Unbundle By Name(w93) -> ("Set #"=w95:u32)
              n22 = Greater Or Equal?(x=w95, y=u32 5) -> (x >= y?=w96:bool)
            }
            frame True {
              n23 = global read "Global Variables.vi" "Timer Elapsed"() -> (w102:bool)
              n24 = global read "Global Variables.vi" "Abort Scan"() -> (w104:bool)
              n25 = Or(x=w102, y=w104) -> (x .or. y?=w103:bool)
              n26 = case shown="True" w103 {
                tunnel: w108 -> [w113 w119]
                tunnel: w107 -> [_ w120]
                tunnel: [w113 w118] -> w106
                tunnel: [errorcluster {"status"=FALSE, "code"=0, "source"=""} ("error out") w117] -> w105
                tunnel: [w112 w116] -> w101
                tunnel: w100 -> [_ w115]
                frame False {
                  n27 = Unbundle By Name(w113) -> ("Magnet Angle [deg]"=w112:dbl)
                }
                frame True {
                  n28 = stacked-sequence {
                    tunnel: w120 -> [_ w127]
                    tunnel: w119 -> [_ w126]
                    tunnel: [_ w125] -> w118
                    tunnel: [_ w124] -> w117
                    tunnel: [_ w123] -> w116
                    tunnel: w115 -> [w121 _]
                    frame #0 {
                      n29 = case shown="True" w121 {
                        frame False {
                        }
                        frame True {
                          n30 = One Button Dialog(message="Please remove the subject from the magnet, and click OK") -> ()  [unwired: 1 in, 1 out]
                        }
                      }
                    }
                    frame #1 {
                      w123 = 0.0 ("Magnet Angle [deg]")
                      n31 = Bundle By Name(cluster=w126, "Magnet Angle [deg]"=w123) -> (w125:T5)
                      n32 = call "Magnet Rotation.vi"("Hardware Parameters"=w127, "Acquisition Parameters"=w125) -> ("error out"=w124:errorcluster)  [unwired: 8 in, 1 out]
                    }
                  }
                }
              }
              n33 = Select(t=cluster{"Enum":T4, "Data":variant}[] [{"Enum"=enum."End Session", "Data"=variant}], s=w103, f=cluster{"Enum":T4, "Data":variant}[] [{"Enum"=enum."Configure Hardware", "Data"=variant}, {"Enum"=enum."Initialize Set", "Data"=variant}, {"Enum"=enum."Read GUI Pars", "Data"=variant}, {"Enum"=enum."Pre-Scan", "Data"=variant}]) -> (s? t:f=w109:cluster{"Enum":T4, "Data":variant}[])
            }
          }
          n34 = case shown="False" w60 {
            frame False {
            }
            frame True {
              n35 = global write "Global Variables.vi" "Popup to Display"("Measurement Complete" ("Message to Display")) -> ()
              n36 = global write "Global Variables.vi" "Display Popup"(TRUE ("Display Popup")) -> ()
            }
          }
          n37 = call "Decision to Report Dose.vi"("Timer Elapsed or Sets # Reached?"=w60, "Measurement Information"=w51, "Acquisition Parameters"=w54) -> ("Report for Adaptive?"=w62:bool, "Report Dose?"=w63:bool)  [unwired: 7 in]
          n38 = case shown="True" w63 {
            tunnel: w51 -> [_ w91]
            tunnel: w69 -> [_ w90]
            frame False {
            }
            frame True {
              n39 = call "Report Dose Measurement Results.vi"("Spectral Data"=w90, "Measurement Information"=w91) -> ()  [unwired: 10 in]
            }
          }
          n40 = case shown="True" w62 {
            tunnel: w72 -> [w79 w87]
            tunnel: [w79 w86] -> w71
            tunnel: w70 -> [w78 w84]
            tunnel: w51 -> [_ w81]
            tunnel: w69 -> [_ w82]
            tunnel: [w78 w83] -> w68
            frame False {
            }
            frame True {
              n41 = call "Check Adaptive - Set.vi"("Spectral Data In"=w82, "Measurement Information In"=w81, "Acquisition Parameters In"=w84) -> ("Set-level Convergence?"=w80:bool, "Acquisition Parameters Out"=w83:T5)  [unwired: 7 in]
              n42 = case shown="True" w80 {
                tunnel: w82 -> [_ w89]
                tunnel: w81 -> [_ w88]
                frame False {
                }
                frame True {
                  n43 = call "Report Dose Measurement Results.vi"("Spectral Data"=w89, "Measurement Information"=w88) -> ()  [unwired: 10 in]
                }
              }
              n44 = Select(t=cluster{"Enum":T4, "Data":variant}[] [{"Enum"=enum."End Session", "Data"=variant}], s=w80, f=w87) -> (s? t:f=w86:cluster{"Enum":T4, "Data":variant}[])
            }
          }
        }
        frame "Oximetry" {
          n45 = Unbundle By Name(w130) -> ("Prompt for oxy acquisition updates"=w145:bool)
          n46 = case shown="True" w145 {
            tunnel: w130 -> [w207 w211]
            tunnel: w146 -> [_ w210]
            tunnel: w141 -> [_ w209]
            tunnel: [w207 w208] -> w133
            frame False {
            }
            frame True {
              n47 = call "Prompt for Oximetry Acquisition Updates-Rev2.vi"("Spectral Data In"=w209, "Hardware Parameters In"=w210, "Acquisition Parameters In"=w211) -> ("Acquisition Parameters Out"=w208:T5)  [unwired: 8 in]
            }
          }
          n48 = Unbundle By Name(w135) -> ("Save Data"=w134:bool)
          n49 = case shown="True" w134 {
            tunnel: w135 -> [w147 w154]
            tunnel: w141 -> [_ w151]
            tunnel: [w148 w158] -> w138
            tunnel: [w149 w157] -> w137
            tunnel: [w147 w153] -> w129
            tunnel: w130 -> [_ w152]
            tunnel: [_ w150] -> w128
            frame False {
              n50 = Unbundle By Name(w147) -> ("Linewidth (HWHM)/Set [Gauss]"=w149:dbl[][], "pO2/Set [mmHg]"=w148:dbl[][])
            }
            frame True {
              n51 = call "Report Oximetry Set-Rev1.vi"("Spectral Data In"=w151, "Measurement Information In"=w154, "Acquisition Parameters In"=w152) -> ("Report pO2"=w156:bool, "Measurement Information Out"=w155:T1)  [unwired: 7 in]
              n52 = case shown="True" w156 {
                tunnel: w155 -> [w159 w163]
                tunnel: [dbl[][] [] ("pO2/Set [mmHg]") w171] -> w158
                tunnel: [w160 dbl[][] [] ("Calibration dBpp/Set [Gauss]")] -> w157
                tunnel: [w159 w167] -> w153
                tunnel: w152 -> [_ w165]
                tunnel: w151 -> [_ w164]
                tunnel: [_ w162] -> w150
                frame False {
                  n53 = Unbundle By Name(w159) -> ("Linewidth (HWHM)/Set [Gauss]"=w160:dbl[][])
                }
                frame True {
                  n54 = Unbundle By Name(w163) -> ("Report pO2/Scan"=w169:bool, "Oxy Exclude Unacceptable"=w168:bool, "Oxy Unacceptable Estimate Flags"=w166:bool[])
                  n55 = Unbundle By Name(w163) -> ("pO2/Set [mmHg]"=w171:dbl[][])
                  n56 = case shown="False" w169 {
                    tunnel: w168 -> [w178 _]
                    tunnel: [w177 w190] -> w167
                    tunnel: w166 -> [w176 _]
                    tunnel: w163 -> [w175 w190]
                    tunnel: w165 -> [w174 _]
                    tunnel: w164 -> [w173 _]
                    tunnel: [w172 _] -> w162
                    frame False {
                      n57 = case shown="True" w178 {
                        tunnel: [w179 w189] -> w177
                        tunnel: w176 -> [_ w188]
                        tunnel: w175 -> [w179 w184]
                        tunnel: w174 -> [_ w186]
                        tunnel: w173 -> [_ w185]
                        tunnel: [_ w180] -> w172
                        frame False {
                        }
                        frame True {
                          n58 = Unbundle By Name(w184) -> ("Set #"=w183:u32)
                          n59 = call "Exclude pO2 Estimate-Rev2.vi"("Spectral Data In"=w185, "Measurement Information In"=w184, "Acquisition Parameters In"=w186) -> ("Exclude pO2 Estimate"=w180:bool)  [unwired: 8 in]
                          n60 = Decrement(x=w183) -> (x-1=w182:u32)
                          n61 = To Long Integer(number=w182) -> (32bit integer=w181:i32)
                          n62 = Insert Into Array(array=w188, index=w181, new element=w180) -> (w187:bool[])
                          n63 = Bundle By Name(cluster=w184, "Oxy Unacceptable Estimate Flags"=w187) -> (w189:T1)
                        }
                      }
                    }
                    frame True {
                    }
                  }
                }
              }
            }
          }
          n64 = Unbundle By Name(w133) -> ("Oxy QA Scan?"=w144:bool, "Optimizing RF Power"=w143:bool)
          n65 = case shown="False" w144 {
            tunnel: [w196 cluster{"Enum":T4, "Data":variant}[] [{"Enum"=enum."Read GUI Pars", "Data"=variant}, {"Enum"=enum."Idle", "Data"=variant}]] -> w142
            tunnel: w133 -> [w191 w201]
            tunnel: [w194 w204] -> w139
            tunnel: w143 -> [w195 _]
            tunnel: [w193 w203] -> w132
            tunnel: [w192 w202] -> w131
            frame False {
              n66 = case shown="False" w195 {
                tunnel: [cluster{"Enum":T4, "Data":variant}[] [{"Enum"=enum."Idle", "Data"=variant}] cluster{"Enum":T4, "Data":variant}[] [{"Enum"=enum."Optimize RF Power", "Data"=variant}, {"Enum"=enum."Idle", "Data"=variant}]] -> w196
                tunnel: w191 -> [w197 w199]
                tunnel: [w197 w199] -> w194
                frame False {
                }
                frame True {
                }
              }
              n67 = Unbundle By Name(w191) -> ("Scan Width [G]"=w193:dbl, "Mod. Amp. [G]"=w192:dbl)
            }
            frame True {
              n68 = Unbundle By Name(w201) -> ("OxyQAInit Scan Width [G]"=w203:dbl, "OxyQAInit Mod. Amp. [G]"=w202:dbl)
              n69 = Bundle By Name(cluster=w201, "Oxy QA Scan?"=FALSE, "Scan Width [G]"=w203, "Mod. Amp. [G]"=w202) -> (w204:T5)
            }
          }
        }
      }
    }
    frame True {
      n70 = Unbundle By Name(w212) -> ("Linewidth (HWHM)/Set [Gauss]"=w228:dbl[][], "pO2/Set [mmHg]"=w229:dbl[][])
      n71 = Unbundle By Name(w223) -> ("First CheckCal Scan?"=w225:bool, "Scan Width [G]"=w214:dbl, "Mod. Amp. [G]"=w213:dbl)
      n72 = Equal?(x=enum16{"Engineering", "Dosimetry", "Oximetry"}."Dosimetry" ("DAQ Mode"), y=w219) -> (x = y?=w217:bool)
      n73 = Unbundle By Name(w212) -> ("QA Mode"=w227:T9)
      n74 = case shown="True" w217 {
        tunnel: w216 -> [w230 w233]
        tunnel: w212 -> [_ w232]
        tunnel: [w230 w231] -> w215
        frame False {
        }
        frame True {
          n75 = call "Append to PDT and Tooth History.vi"("Spectral Data In"=w233, "Measurement Information In"=w232) -> ("Spectral Data Out"=w231:T6)  [unwired: 9 in]
        }
      }
      n76 = case shown="\"QA-Start/End\"..\"QA-Weekly\"" w227 {
        tunnel: [cluster{"Enum":T4, "Data":variant}[] [{"Enum"=enum."Idle", "Data"=variant}] w238 cluster{"Enum":T4, "Data":variant}[] [{"Enum"=enum."Idle", "Data"=variant}] w285] -> w226
        tunnel: w225 -> [_ _ _ w287]
        tunnel: w223 -> [w234 w241 w280 w283]
        tunnel: w224 -> [_ w240 _ _]
        tunnel: w212 -> [_ w243 _ _]
        tunnel: [w234 w242 w280 w283] -> w222
        tunnel: [w235 w239 w279 w282] -> w220
        tunnel: [_ w237 _ _] -> w221
        frame "Select QA Mode", Default {
          n77 = Unbundle By Name(w234) -> ("Magnet Angle [deg]"=w235:dbl)
        }
        frame "QA-Start/End".."QA-Weekly" {
          n78 = Unbundle By Name(w240) -> ("Magnet Rotation"=w244:bool)
          n79 = Unbundle By Name(w241) -> ("Running Script"=w246:bool)
          n80 = Not(x=w246) -> (.not. x?=w245:bool)
          n81 = And(x=w244, y=w245) -> (x .and. y?=w247:bool)
          n82 = case shown="False" w247 {
            tunnel: w241 -> [w254 w269]
            tunnel: w240 -> [_ w268]
            tunnel: [w254 w267] -> w242
            tunnel: [_ w266] -> w237
            tunnel: w243 -> [w251 _]
            tunnel: [0.0 ("Magnet Angle [deg]") w264] -> w239
            tunnel: [w248 w260] -> w238
            frame False {
              n83 = Unbundle By Name(w251) -> ("Set #"=w253:u32)
              n84 = Greater Or Equal?(x=w253, y=u32 5) -> (x >= y?=w249:bool)
              n85 = case shown="False" w249 {
                tunnel: [w255 cluster{"Enum":T4, "Data":variant}[] [{"Enum"=enum."End Session", "Data"=variant}, {"Enum"=enum."New Session", "Data"=variant}]] -> w248
                frame False {
                  n86 = flat-sequence {
                    tunnel: [cluster{"Enum":T4, "Data":variant}[] [{"Enum"=enum."Configure Hardware", "Data"=variant}, {"Enum"=enum."Initialize Set", "Data"=variant}, {"Enum"=enum."Read GUI Pars", "Data"=variant}, {"Enum"=enum."Pre-Scan", "Data"=variant}]] -> w255
                    frame #0 {
                      n87 = One Button Dialog(message="Please replace the resonator on the sample, and then click OK.") -> ()  [unwired: 1 in, 1 out]
                    }
                    frame #1 {
                    }
                  }
                }
                frame True {
                }
              }
            }
            frame True {
              n88 = global read "Global Variables.vi" "Timer Elapsed"() -> (w263:bool)
              n89 = global read "Global Variables.vi" "Abort Scan"() -> (w265:bool)
              n90 = Or(x=w263, y=w265) -> (x .or. y?=w259:bool)
              n91 = case shown="True" w259 {
                tunnel: w269 -> [w273 w277]
                tunnel: w268 -> [_ w278]
                tunnel: [w273 w276] -> w267
                tunnel: [_ w275] -> w266
                tunnel: [w272 w274] -> w264
                frame False {
                  n92 = Unbundle By Name(w273) -> ("Magnet Angle [deg]"=w272:dbl)
                }
                frame True {
                  w274 = 0.0 ("Magnet Angle [deg]")
                  n93 = Bundle By Name(cluster=w277, "Magnet Angle [deg]"=w274) -> (w276:T5)
                  n94 = call "Magnet Rotation.vi"("Hardware Parameters"=w278, "Acquisition Parameters"=w276) -> ("error out"=w275:errorcluster)  [unwired: 8 in, 1 out]
                }
              }
              n95 = case shown="True" w263 {
                frame False {
                }
                frame True {
                  n96 = global write "Global Variables.vi" "Display Popup"(TRUE ("Display Popup")) -> ()
                  n97 = global write "Global Variables.vi" "Popup to Display"("Measurement Complete" ("Message to Display")) -> ()
                }
              }
              n98 = Select(t=cluster{"Enum":T4, "Data":variant}[] [{"Enum"=enum."End Session", "Data"=variant}, {"Enum"=enum."New Session", "Data"=variant}], s=w259, f=cluster{"Enum":T4, "Data":variant}[] [{"Enum"=enum."Configure Hardware", "Data"=variant}, {"Enum"=enum."Initialize Set", "Data"=variant}, {"Enum"=enum."Pre-Scan", "Data"=variant}]) -> (s? t:f=w260:cluster{"Enum":T4, "Data":variant}[])
            }
          }
        }
        frame "QA-Eng" {
          n99 = Unbundle By Name(w280) -> ("Magnet Angle [deg]"=w279:dbl)
        }
        frame "Check Calibration" {
          n100 = Unbundle By Name(w283) -> ("Magnet Angle [deg]"=w282:dbl)
          n101 = Select(t=cluster{"Enum":T4, "Data":variant}[] [], s=w287, f=cluster{"Enum":T4, "Data":variant}[] [{"Enum"=enum."Check Calibration", "Data"=variant}]) -> (s? t:f=w285:cluster{"Enum":T4, "Data":variant}[])
        }
      }
    }
  }
  "Spectral Data Out" <- w16
  "Acquisition Parameters Out" <- w17
  "QSM Response" <- w15
  "pO2/Set [mmHg]" <- w14
  "Calibration dBpp/Set [Gauss]" <- w13
  "Magnet Angle [deg]" <- w12
  "error out" <- w11
  "Scan Width [G]" <- w9
  "Mod. Amp. [G]" <- w8
  "Measurement Information Out" <- w7
  "Exclude pO2 Estimate" <- w1
